vi "Explorer.vi"(11 "String in":refnum<vi>) -> ()   [LabVIEW 2020]
panel:
  in  "Tab Control":enum32{"Scope", "Gauges"}(tab)
  out "Graph":dbl[][](graph)
  in  "Clear":bool
  out "Data":dbl[](array[knob]) scale=-100.0..100.0
  out "New line":bool
  out "Value":string
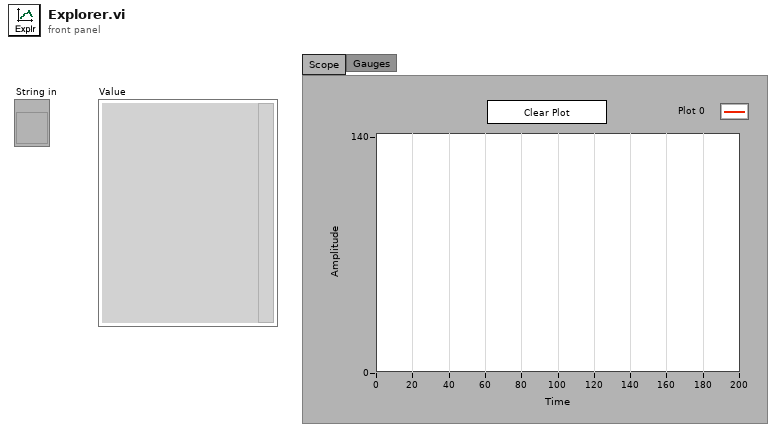
[diagram p1: front panel]
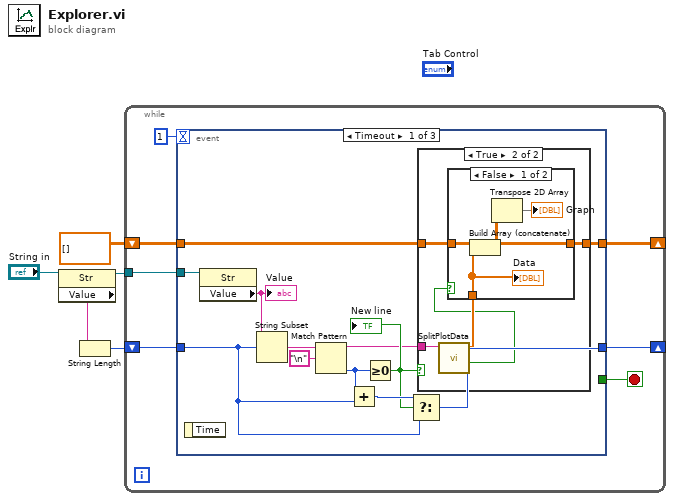
[diagram p0: block diagram]
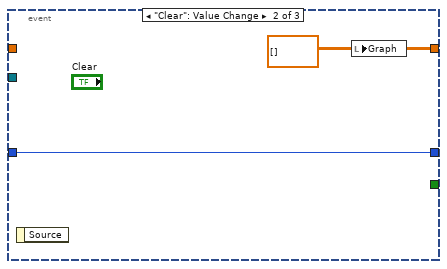
[diagram p4: hidden frame]
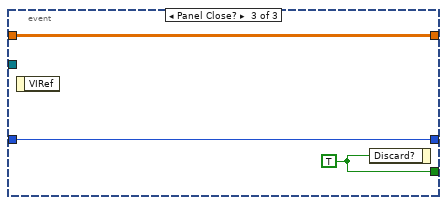
[diagram p5: hidden frame]
diagram:
  n1 = property class="Str"(reference="String in") -> (reference out=w2:refnum<vi>, "Value"=w4:string)  [unwired: 1 in, 1 out]
  n2 = String Length(string=w4) -> (length=w5:i32)
  n3 = while {
    tunnel: w2 -> [w10]
    shift-right: [w9] -> _
    shift-left: w5 -> [w8]
    shift-right: [w6] -> _
    shift-left: dbl[][] [] -> [w7]
    stop <- w11 stop-if-true
    n4 = event shown="[0] Timeout" {
      selector: _ -> [_ _ _]
      dyn-events: _ -> [_ _ _]
      timeout: 1 -> [_ _ _]
      tunnel: [_ _ w40] -> w11
      tunnel: w10 -> [w24 _ _]
      tunnel: [w20 w37 w39] -> w9
      tunnel: w8 -> [w18 w37 w39]
      tunnel: w7 -> [w14 _ w38]
      tunnel: [w13 w36 w38] -> w6
      event Timeout {
        n5 = event-data() -> ()  [unwired: 1 in, 1 out]
        n6 = property class="Str"(reference=w24) -> ("Value"=w23:string)  [unwired: 1 in, 2 out]
        "Value" <- w23
        n7 = String Subset(string=w23, offset (0)=w18) -> (substring=w22:string)  [unwired: 1 in]
        n8 = Match Pattern(string=w22, regular expression="\n") -> (before substring=w15:string, offset past match=w19:i32)  [unwired: 1 in, 2 out]
        n9 = Add(x=w19, y=w18) -> (x+y=w17:i32)
        n10 = Greater Or Equal To 0?(x=w19) -> (x >= 0?=w16:bool)
        "New line" <- w16
        n11 = Select(t=w17, s=w16, f=w18) -> (s? t:f=w20:i32)
        n12 = case shown="True" w16 {
          tunnel: w15 -> [_ w30]
          tunnel: w14 -> [w25 w29]
          tunnel: [w25 w27] -> w13
          frame False {
          }
          frame True {
            n13 = call "SplitPlotData.vi"("Value"=w30) -> ("not a number"=w26:bool, "Array"=w28:dbl[])  [unwired: 9 in]
            n14 = case shown="False" w26 {
              tunnel: w29 -> [w34 w35]
              tunnel: w28 -> [w31 _]
              tunnel: [w33 w35] -> w27
              frame False {
                n15 = Build Array (concatenate)(w34, w31) -> (w33:dbl[][])
                n16 = Transpose 2D Array(2D array=w33) -> (transposed array=→"Graph":dbl[][])
                "Data" <- w31
              }
              frame True {
              }
            }
          }
        }
      }
      event "Clear": Value Change {
        w36 = dbl[][] []
        n17 = event-data() -> ()  [unwired: 1 in, 1 out]
        n18 = local write "Graph"(w36) -> ()
      }
      event Panel Close? {
        w40 = TRUE ("Discard?")
        n19 = event-data() -> ()  [unwired: 1 in, 1 out]
        n20 = event-data("Discard?"=w40) -> ()  [unwired: 1 in, 1 out]
      }
    }
  }
